vi "RemoveAllNames.vi"(11 "Names":string[](array[string])) -> ()   [LabVIEW 2014]
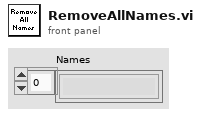
[diagram p1: front panel]
types:
  T1 = enum16{"New", "Find", "FindPattern", "GetTable", "Clear"}
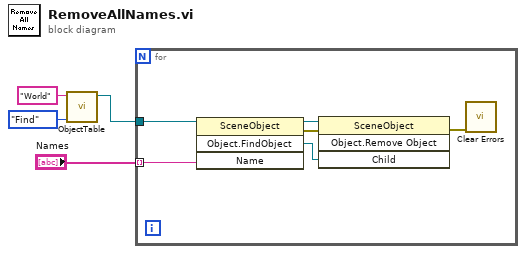
[diagram p0: block diagram]
diagram:
  n1 = call "ObjectTable.vi"("ObjectStoreSelector"=T1."Find", "Name"="World") -> ("ObjectRef"=w1:refnum<vi>)  [unwired: 5 in, 4 out]
  n2 = for {
    tunnel: "Names" -> [w7] mode=indexing
    tunnel: w1 -> [w6]
    n3 = invoke class="SceneObject" method="Object.FindObject"(reference=w6, "Name"=w7) -> (reference out=w10:refnum<vi>, error out=w8:errorcluster, "FindObject"=w9:refnum<vi>)  [unwired: 2 in, 1 out]
    n4 = invoke class="SceneObject" method="Object.Remove Object"(reference=w10, error in=w8, "Child"=w9) -> (error out=w5:errorcluster)  [unwired: 1 in, 3 out]
    n5 = call <vilib>:"Clear Errors.vi"("error in (no error)"=w5) -> ()  [unwired: 5 in, 2 out]
  }
